vi "Parse Structure Recursive with Fast Tree.vi"(8 "error in":errorcluster, 10 "Node":T1, 11 "ParseGDSII in":refnum<class "ParseGDSII.lvclass">) -> (0 "error out":errorcluster, 2 "Geometric":refnum<class "Geometric.lvclass">[](array[class]), 3 "ParseGDSII out":refnum<class "ParseGDSII.lvclass">)   [LabVIEW 2019, in "ParseGDSII.lvclass"]
uses:
  ParseGDSII.lvclass
  Elements/Geometric.lvclass
  C:/Users/Albro/Documents/GitHub/AFM-Lithography/lvsrc/Classes/Parse/GDSII/Elements/Element.lvclass
  Elements/Referential.lvclass
  ParseGDSII.lvclass/ParseGDSII.ctl
  Fast Tree/Fast Tree.lvclass
  Elements/Element.lvclass
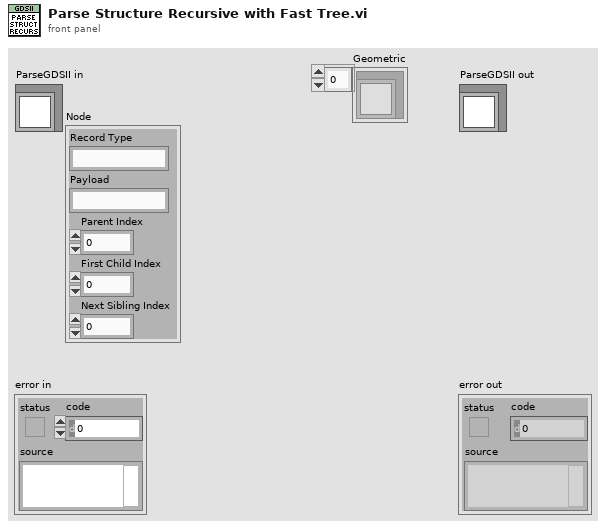
[diagram p1: front panel]
types:
  T1 = cluster{"Record Type":string, "Payload":string, "Parent Index":i32, "First Child Index":i32, "Next Sibling Index":i32}
  T2 = cluster{"Record Type":string, "Payload":string, "Parent Index":i32, "First Child Index":i32, "Next Sibling Index":i32}[]
  T3 = typedef "NI_Matrix.lvlib/RealMatrix.ctl" = dbl[][]
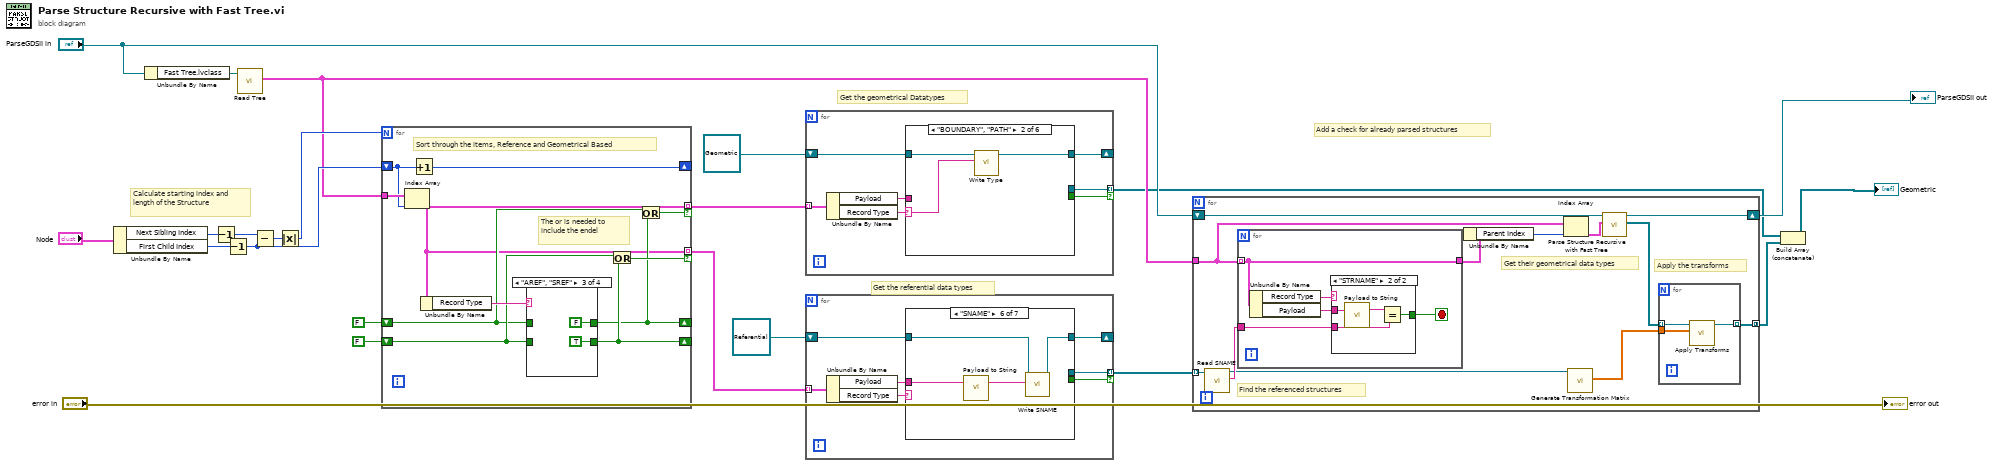
[diagram p0: block diagram]
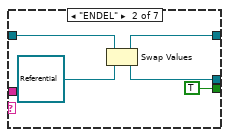
[diagram p4: hidden frame]
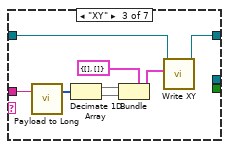
[diagram p5: hidden frame]
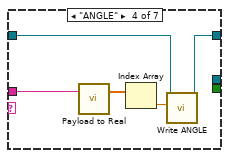
[diagram p6: hidden frame]
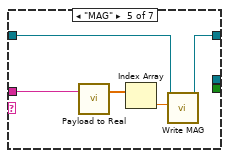
[diagram p7: hidden frame]
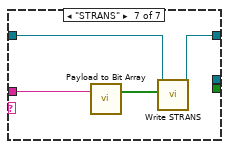
[diagram p8: hidden frame]
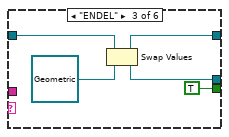
[diagram p10: hidden frame]
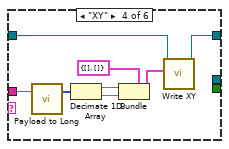
[diagram p11: hidden frame]
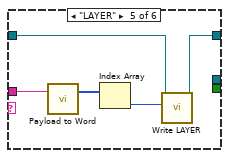
[diagram p12: hidden frame]
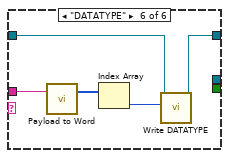
[diagram p13: hidden frame]
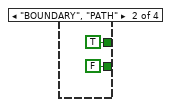
[diagram p15: hidden frame]
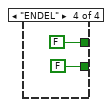
[diagram p16: hidden frame]
diagram:
  # "Add a check for already parsed structures"
  # "Get the referential data types"
  # "Get the geometrical Datatypes"
  # "Calculate starting index and length of the Structure"
  n1 = Unbundle By Name("Node") -> ("Next Sibling Index"=w14:i32, "First Child Index"=w13:i32)
  n2 = Unbundle By Name("ParseGDSII in") -> ("Fast Tree.lvclass"=w4:refnum<class "Fast Tree.lvclass">)
  n3 = Decrement(x=w14) -> (x-1=w12:i32)
  n4 = Decrement(x=w13) -> (x-1=w9:i32)
  n5 = call-dynamic "Read Tree.vi"("Fast Tree in"=w4) -> ("Tree"=w3:T2)  [unwired: 8 in, 2 out]
  n6 = Subtract(x=w12, y=w9) -> (x-y=w11:i32)
  n7 = Absolute Value(x=w11) -> (abs(x)=w10:i32)
  n8 = for {
    N: w10 -> [_]
    shift-right: [w26] -> _
    shift-left: FALSE -> [w24]
    tunnel: [w23] -> w16 mode=indexing if=w25
    tunnel: w3 -> [w32]
    shift-right: [w30] -> _
    shift-left: w9 -> [w31]
    shift-right: [w29] -> _
    shift-left: FALSE -> [w28]
    tunnel: [w23] -> w7 mode=indexing if=w27
    # "The or is needed to include the endel"
    # "Sort through the items, Reference and Geometrical Based"
    n9 = Index Array(array=w32, index=w31) -> (element=w23:T1)
    n10 = Increment(x=w31) -> (x+1=w30:i32)
    n11 = Unbundle By Name(w23) -> ("Record Type"=w33:string)
    n12 = case shown="\"AREF\", \"SREF\"" w33 {
      tunnel: [w35 TRUE FALSE FALSE] -> w26
      tunnel: w24 -> [w35 _ _ _]
      tunnel: [w34 FALSE TRUE FALSE] -> w29
      tunnel: w28 -> [w34 _ _ _]
      frame Default {
      }
      frame "BOUNDARY", "PATH" {
      }
      frame "AREF", "SREF" {
      }
      frame "ENDEL" {
      }
    }
    n13 = Or(x=w28, y=w29) -> (x .or. y?=w27:bool)
    n14 = Or(x=w24, y=w26) -> (x .or. y?=w25:bool)
  }
  n15 = for {
    tunnel: w16 -> [w48] mode=indexing
    tunnel: [w43] -> w1 mode=indexing if=w42
    shift-right: [w45] -> _
    shift-left: refnum<class "Geometric.lvclass"> refnum ("Element out") -> [w44]
    n16 = Unbundle By Name(w48) -> ("Payload"=w47:string, "Record Type"=w46:string)
    n17 = case shown="\"BOUNDARY\", \"PATH\"" w46 {
      selector: w46 -> [_ w50 _ _ _ _]
      tunnel: w47 -> [_ _ _ w60 w68 w74]
      tunnel: [w49 w52 w53 w59 w66 w72] -> w45
      tunnel: w44 -> [w49 w51 w54 w58 w67 w73]
      tunnel: [_ _ w55 _ _ _] -> w43
      tunnel: [_ _ TRUE _ _ _] -> w42
      frame Default {
      }
      frame "BOUNDARY", "PATH" {
        n18 = call-dynamic "Write Type.vi"("Type"=w50, "Element in"=w51) -> ("Element out"=w52:refnum<class "Geometric.lvclass">)  [unwired: 8 in, 1 out]
      }
      frame "ENDEL" {
        n19 = Swap Values(12:w54, 14:refnum<class "Geometric.lvclass"> refnum ("Element out")) -> (1:w53:refnum<class "Geometric.lvclass">, 3:w55:refnum<class "Geometric.lvclass">)  [unwired: 1 in]
      }
      frame "XY" {
        n20 = call "Payload to Long.vi"("Payload"=w60) -> ("Long"=w63:i32[])  [unwired: 2 in]
        n21 = Decimate 1D Array(w63) -> (w65:i32[], w64:i32[])
        n22 = Bundle(cluster=cluster{"X":i32[], "Y":i32[]} {"X"=[], "Y"=[]} ("XY"), "X"=w65, "Y"=w64) -> (w62:cluster{"X":i32[], "Y":i32[]})
        n23 = call-dynamic "Write XY.vi"("XY"=w62, "Element in"=w58) -> ("Element out"=w59:refnum<class "Geometric.lvclass">)  [unwired: 8 in, 1 out]
      }
      frame "LAYER" {
        n24 = call "Payload to Word.vi"("Payload"=w68) -> ("Word"=w69:i16[])  [unwired: 2 in]
        n25 = Index Array(array=w69) -> (element=w70:i16)  [unwired: 1 in]
        n26 = call-dynamic "Write LAYER.vi"("LAYER"=w70, "Geometric in"=w67) -> ("Geometric out"=w66:refnum<class "Geometric.lvclass">)  [unwired: 8 in, 1 out]
      }
      frame "DATATYPE" {
        n27 = call "Payload to Word.vi"("Payload"=w74) -> ("Word"=w75:i16[])  [unwired: 2 in]
        n28 = Index Array(array=w75) -> (element=w71:i16)  [unwired: 1 in]
        n29 = call-dynamic "Write DATATYPE.vi"("DATATYPE"=w71, "Geometric in"=w73) -> ("Geometric out"=w72:refnum<class "Geometric.lvclass">)  [unwired: 8 in, 1 out]
      }
    }
  }
  n30 = for {
    tunnel: w7 -> [w82] mode=indexing
    tunnel: [w77] -> w5 mode=indexing if=w76
    shift-right: [w79] -> _
    shift-left: refnum<class "Referential.lvclass"> refnum ("Referential.lvclass") -> [w78]
    n31 = Unbundle By Name(w82) -> ("Payload"=w81:string, "Record Type"=w80:string)
    n32 = case shown="\"SNAME\"" w80 {
      tunnel: w81 -> [_ _ w91 w97 w105 w108 w111]
      tunnel: [w83 w85 w90 w100 w103 w110 w113] -> w79
      tunnel: w78 -> [w83 w86 w89 w101 w104 w109 w114]
      tunnel: [_ w87 _ _ _ _ _] -> w77
      tunnel: [_ TRUE _ _ _ _ _] -> w76
      frame Default {
      }
      frame "ENDEL" {
        n33 = Swap Values(12:w86, 14:refnum<class "Referential.lvclass"> refnum ("Referential.lvclass")) -> (1:w85:refnum<class "Referential.lvclass">, 3:w87:refnum<class "Referential.lvclass">)  [unwired: 1 in]
      }
      frame "XY" {
        n34 = call "Payload to Long.vi"("Payload"=w91) -> ("Long"=w94:i32[])  [unwired: 2 in]
        n35 = Decimate 1D Array(w94) -> (w96:i32[], w95:i32[])
        n36 = Bundle(cluster=cluster{"X":i32[], "Y":i32[]} {"X"=[], "Y"=[]} ("XY"), "X"=w96, "Y"=w95) -> (w93:cluster{"X":i32[], "Y":i32[]})
        n37 = call-dynamic "Write XY.vi"("XY"=w93, "Element in"=w89) -> ("Element out"=w90:refnum<class "Referential.lvclass">)  [unwired: 8 in, 1 out]
      }
      frame "ANGLE" {
        n38 = call "Payload to Real.vi"("Payload"=w97) -> ("Real"=w98:dbl[])  [unwired: 2 in]
        n39 = Index Array(array=w98) -> (element=w99:dbl)  [unwired: 1 in]
        n40 = call-dynamic "Write ANGLE.vi"("ANGLE"=w99, "Referential in"=w101) -> ("Referential out"=w100:refnum<class "Referential.lvclass">)  [unwired: 8 in, 1 out]
      }
      frame "MAG" {
        n41 = call "Payload to Real.vi"("Payload"=w105) -> ("Real"=w106:dbl[])  [unwired: 2 in]
        n42 = Index Array(array=w106) -> (element=w102:dbl)  [unwired: 1 in]
        n43 = call-dynamic "Write MAG.vi"("MAG"=w102, "Referential in"=w104) -> ("Referential out"=w103:refnum<class "Referential.lvclass">)  [unwired: 8 in, 1 out]
      }
      frame "SNAME" {
        n44 = call "Payload to String.vi"("Payload"=w108) -> ("String"=w107:string)  [unwired: 2 in]
        n45 = call-dynamic "Write SNAME.vi"("SNAME"=w107, "Referential in"=w109) -> ("Referential out"=w110:refnum<class "Referential.lvclass">)  [unwired: 8 in, 1 out]
      }
      frame "STRANS" {
        n46 = call "Payload to Bit Array.vi"("Payload"=w111) -> ("Bit Array"=w112:bool[])  [unwired: 2 in]
        n47 = call-dynamic "Write STRANS.vi"("STRANS"=w112, "Referential in"=w114) -> ("Referential out"=w113:refnum<class "Referential.lvclass">)  [unwired: 8 in, 1 out]
      }
    }
  }
  n48 = for {
    tunnel: w5 -> [w126] mode=indexing
    tunnel: w3 -> [w119]
    tunnel: [w120] -> w2 mode=concatenating
    shift-right: [w122] -> w18
    shift-left: "ParseGDSII in" -> [w124]
    # "Apply the transforms"
    # "Get their geometrical data types"
    # "Find the referenced structures"
    n49 = call-dynamic "Read SNAME.vi"("Referential in"=w126) -> ("SNAME"=w125:string, "Referential out"=w123:refnum<class "Referential.lvclass">)  [unwired: 8 in, 1 out]
    n50 = for {
      tunnel: w119 -> [w131] mode=indexing
      tunnel: w125 -> [w133]
      tunnel: [w131] -> w118
      stop <- w130 stop-if-true
      n51 = Unbundle By Name(w131) -> ("Record Type"=w134:string, "Payload"=w132:string)
      n52 = case shown="\"STRNAME\"" w134 {
        tunnel: w133 -> [_ w136]
        tunnel: w132 -> [_ w138]
        tunnel: [_ w135] -> w130
        frame "False", Default {
        }
        frame "STRNAME" {
          n53 = call "Payload to String.vi"("Payload"=w138) -> ("String"=w137:string)  [unwired: 2 in]
          n54 = Equal?(x=w137, y=w136) -> (x = y?=w135:bool)
        }
      }
    }
    n55 = Unbundle By Name(w118) -> ("Parent Index"=w117:i32)
    n56 = Index Array(array=w119, index=w117) -> (element=w116:T1)
    n57 = call "Generate Transformation Matrix.vi"("Referential in"=w123) -> ("Matrix"=w115:T3)  [unwired: 8 in, 2 out]
    n58 = call "Parse Structure Recursive with Fast Tree.vi"("Node"=w116, "ParseGDSII in"=w124) -> ("Geometric"=w121:refnum<class "Geometric.lvclass">[], "ParseGDSII out"=w122:refnum<class "ParseGDSII.lvclass">)  [unwired: 7 in, 1 out]
    n59 = for {
      tunnel: w115 -> [w129]
      tunnel: w121 -> [w128] mode=indexing
      tunnel: [w127] -> w120 mode=indexing
      n60 = call "Apply Transforms.vi"("Matrix"=w129, "Element in"=w128) -> ("Element out"=w127:refnum<class "Geometric.lvclass">)  [unwired: 8 in, 1 out]
    }
  }
  "ParseGDSII out" <- w18
  n61 = Build Array (concatenate)(w1, w2) -> (→"Geometric":refnum<class "Geometric.lvclass">[])
  "error out" <- "error in"
